vi "ImageLabview.vi"() -> ()   [LabVIEW 2019]
uses:
  <vilib>/userDefined/High Color/IMAQdx.ctl
  <vilib>/vision/driver/NI_Vision_Acquisition_Software.lvlib
panel:
  in  "stop":bool
  out "Image":T1(plugin-control)
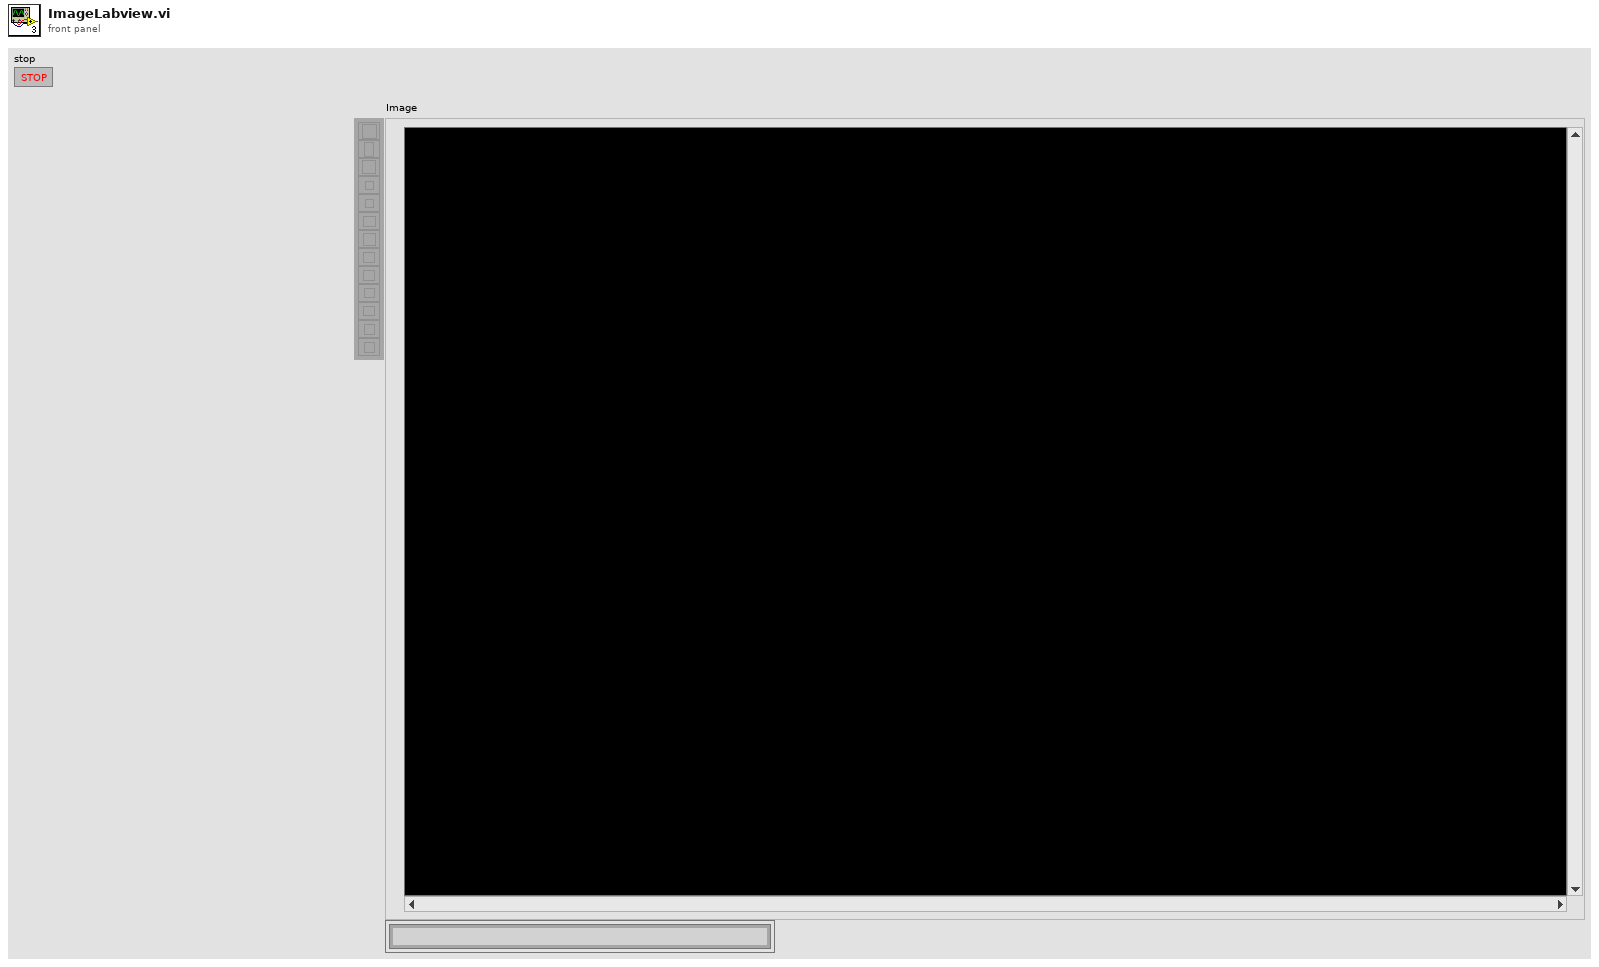
[diagram p1: front panel]
types:
  T1 = typedef "IMAQ Image.ctl" = refnum<image>
  T2 = typedef "IMAQdx.ctl" = refnum<k21>
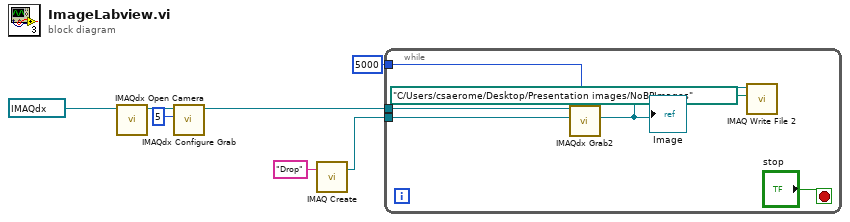
[diagram p0: block diagram]
diagram:
  n1 = call <vilib>:"IMAQdx Open Camera.vi"("Session In"=T2 "cam0") -> ("Session Out"=w7:T2)  [unwired: 9 in, 1 out]
  n2 = call <vilib>:"IMAQdx Configure Grab.vi"("Number of Buffers"=u32 5, "Session In"=w7) -> ("Session Out"=w1:T2)  [unwired: 8 in, 1 out]
  n3 = call "IMAQ Create"("Image Name"="Drop") -> ("New Image"=w2:T1)  [unwired: 4 in, 1 out]
  n4 = while {
    tunnel: 5000 ("Timeout (ms)") -> [w12]
    tunnel: w2 -> [w11]
    tunnel: w1 -> [w10]
    stop <- "stop" stop-if-true
    n5 = call <vilib>:"IMAQdx Grab2.vi"("Timeout (ms)"=w12, "Image In"=w11, "Session In"=w10) -> ("Image Out"=w9:T1)  [unwired: 5 in, 3 out]
    "Image" <- w9
    n6 = call-poly "IMAQ Write File 2"("File Path"=path "C:/Users/csaerome/Desktop/Presentation images/NoBPImages", "Image"=w9) -> ()  [unwired: 8 in, 2 out]
  }
